vi "Instrument.Template.AppLauncher.vi"(8 "error in":errorcluster, 10 "Configuration Window? [T]":bool=TRUE, 11 "Debug Mode? [F]":bool) -> (0 "error out":errorcluster)   [LabVIEW 2019, in "Instrument.Template.lvclass"]
uses:
  Instrument.Template.lvclass
  <vilib>/JKI/JKI SMO/SMO/Typedefs/SMOState --Enum.ctl
  <userlib>/LevyLab/Levylab Instruments/SMOs/Instrument/Instrument.lvclass
  C:/Program Files (x86)/National Instruments/LabVIEW 2019/vi.lib/JKI/JKI SMO/SMO/SMO.lvclass
  <userlib>/LevyLab/Levylab Instruments/SMOs/Instrument UI/Instrument UI.lvclass
  C:/Program Files (x86)/National Instruments/LabVIEW 2019/vi.lib/JKI/JKI SMO/SMO.UI/SMO.UI.lvclass
  Program Files (x86)/National Instruments/LabVIEW 2019/templates/JKI/JKI SMO/Instrument Framework/Templates/Instrument UI.Template/Instrument UI.Template.lvclass
  C:/Program Files (x86)/National Instruments/LabVIEW 2019/user.lib/LevyLab/Levylab Instruments/SMOs/Instrument UI/Instrument UI.lvclass
  C:/Program Files (x86)/National Instruments/LabVIEW 2019/user.lib/LevyLab/Levylab Instruments/SMOs/Instrument/Instrument.lvclass
  <vilib>/JKI/JKI SMO/SMO/SMO.lvclass/SMO.ctl
  <vilib>/JKI/JKI SMO/SMO/Private/ReftoDVR--SMO.vi
  <vilib>/JKI/JKI SMO/SMO/SMO.lvclass
  <vilib>/JKI/JKI SMO/SMO.UI/SMO.UI.lvclass
panel:
  in  "Splash Status":string="Push Start to Start..." caption="String"
  in  "Start":bool=TRUE
  in  "Stop":bool=TRUE
  out "UI SMO State":T1=enum."Stopped"
  out "SMO State":T1
  # "Example Instrument SMO Test Launcher"
  # "For instructions on how to use the JKI State Machine Objects, examples and video tutorials, visit:\nhttp://jki.net/state-machine-objects/\n\nJKI State Machine Objects™\nhttp://jki.net/state-machine-objects/\nCopyright (C) 2005-2015, JKI <info@jki.net>\nALL RIGHTS RESERVED"
  # "Starting Example Instrument..."
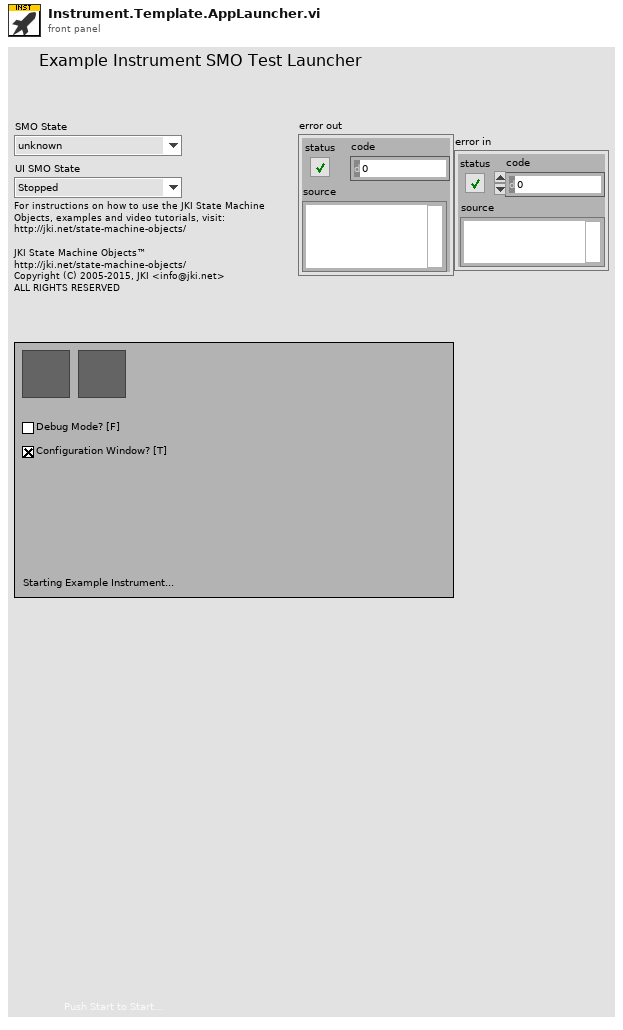
[diagram p1: front panel]
types:
  T1 = typedef "SMO.lvclass/SMOState --Enum.ctl" = enum16{"unknown", "Created", "Started", "Stopped"}
  T2 = enum32{"Invalid", "Standard", "Closed", "Hidden", "Minimized", "Maximized"}
  T3 = enum32{"invalid app kind", "Development System", "Run Time System", "Student Edition", "Embedded LabVIEW", "Evaluation", "Custom"}
  T4 = cluster{"Core":cluster{"Current VI Reference":refnum<vi>, "Close Panel on Exit?":bool}, "Instrument.lvclass":refnum<class "Instrument.lvclass">, "Instrument UI.lvclass":refnum<class "Instrument UI.lvclass">}
  T5 = cluster{"Current VI Reference":refnum<vi>, "Close Panel on Exit?":bool}
  T6 = typedef "SMO.lvclass/Public Events.ctl" = cluster{"Error":refnum<user-event>, "State":refnum<user-event>, "Reserve State":refnum<user-event>}
  T7 = cluster{"Event Registration Refnum":refnum<event-registration>, "Event Registration Refnum":refnum<event-registration>}
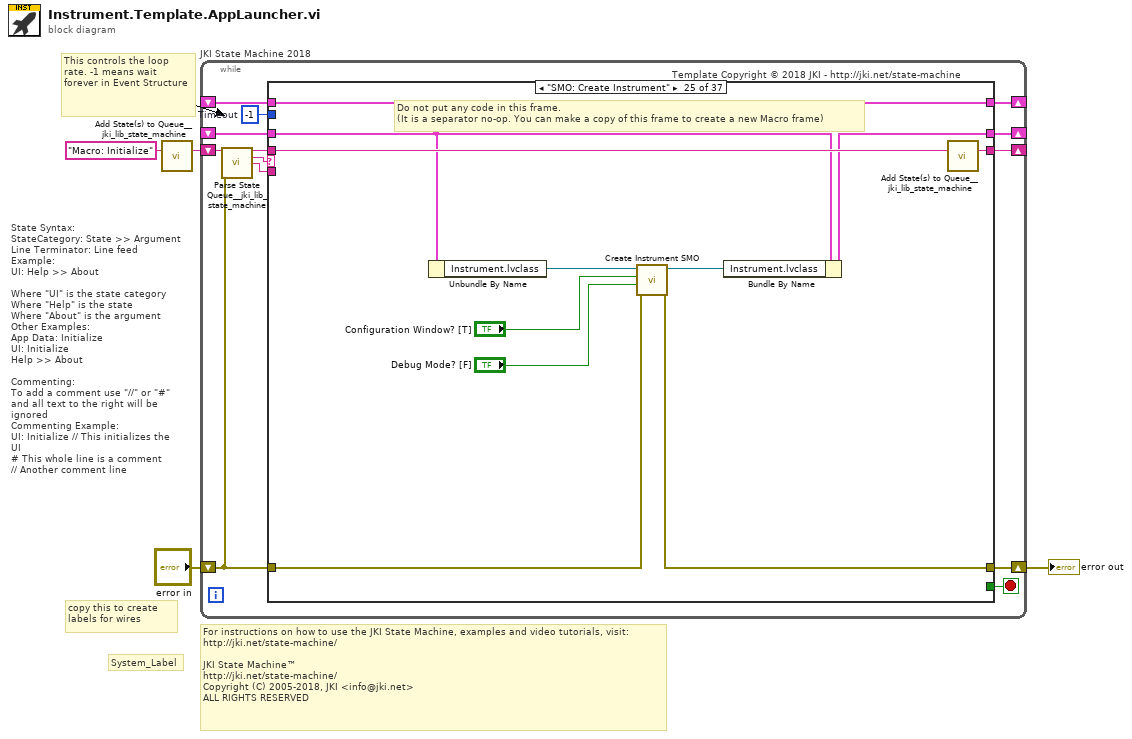
[diagram p0: block diagram]
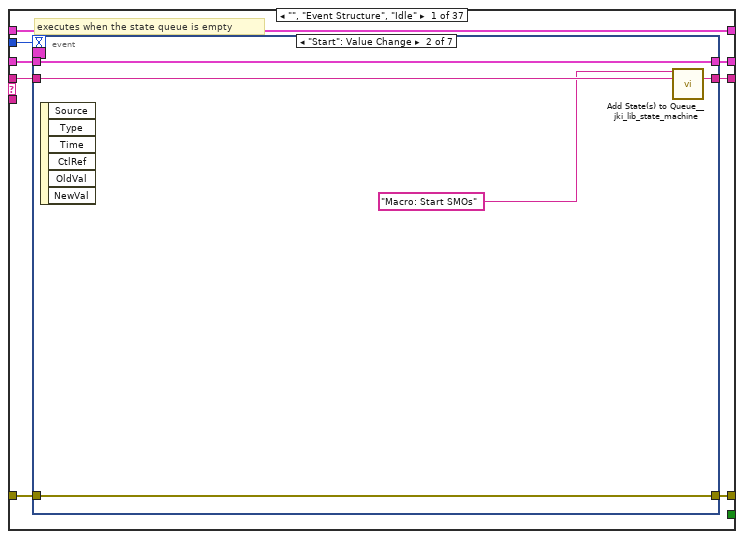
[diagram p2: hidden frame]
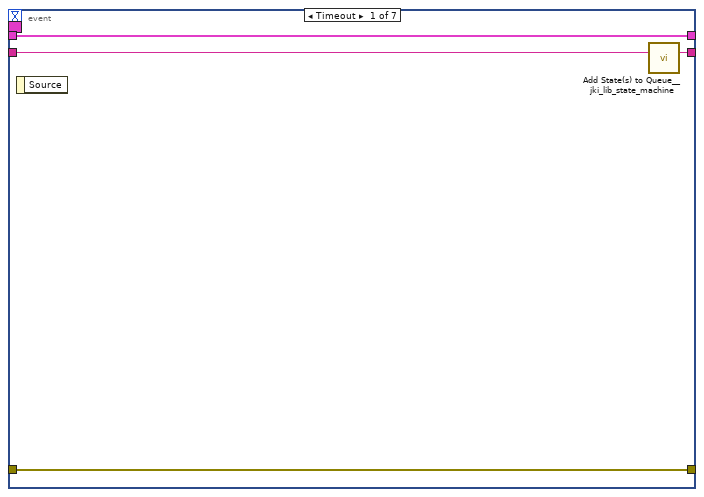
[diagram p3: hidden frame]
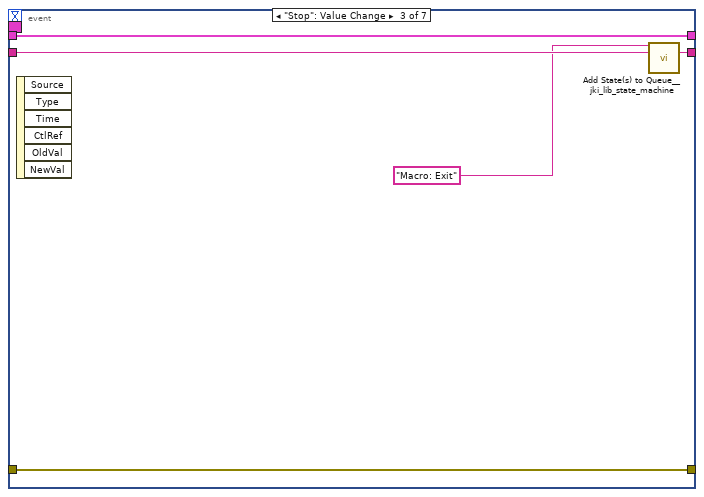
[diagram p4: hidden frame]
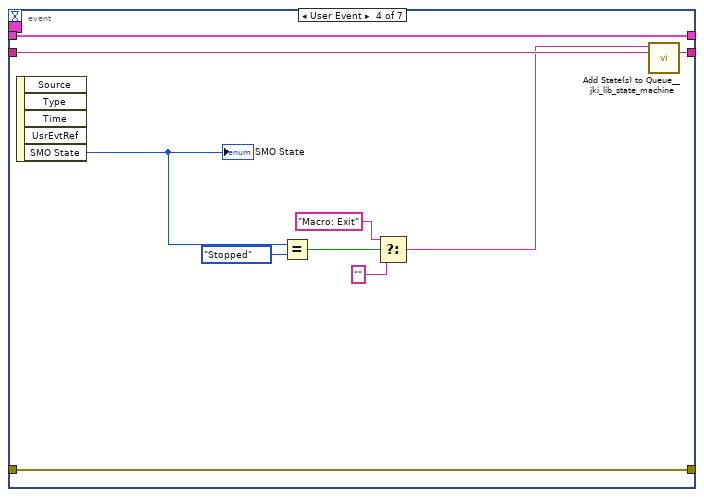
[diagram p5: hidden frame]
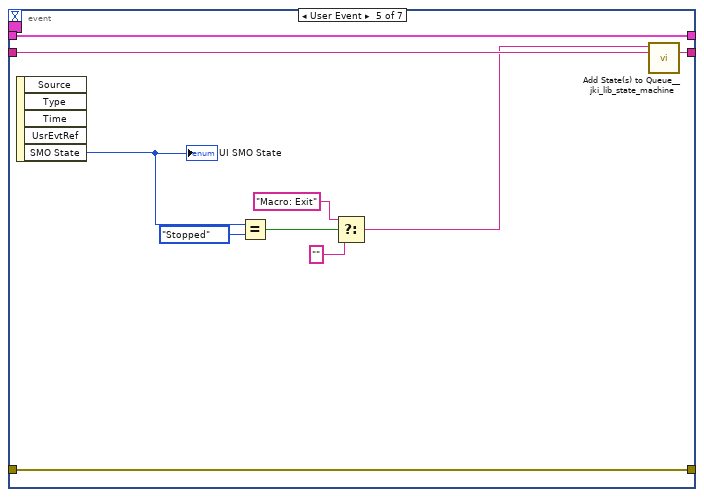
[diagram p6: hidden frame]
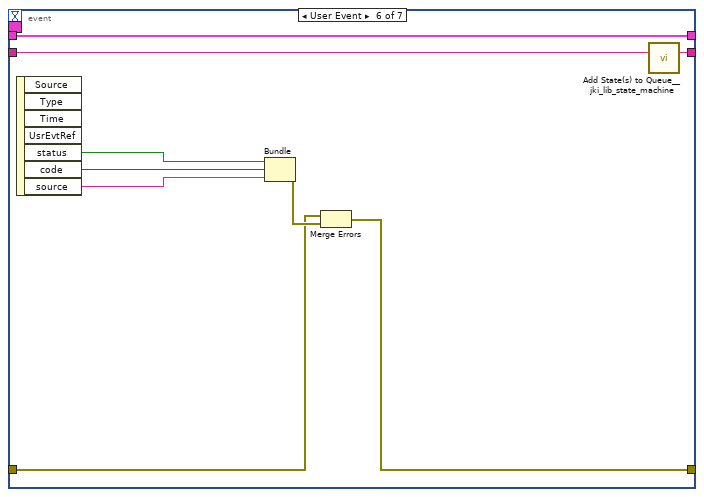
[diagram p7: hidden frame]
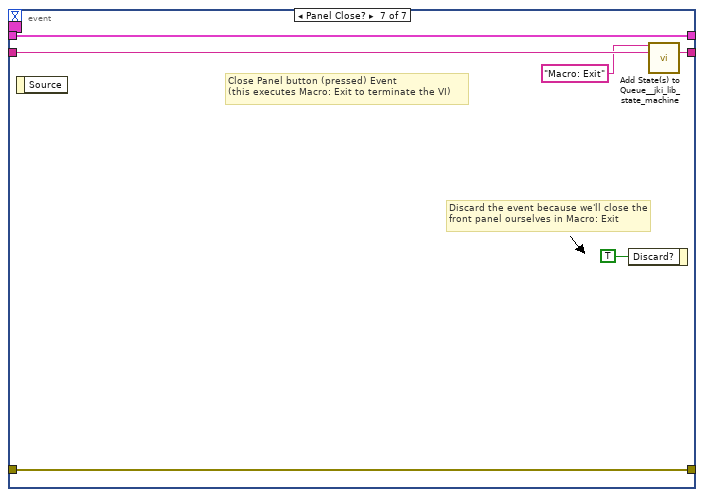
[diagram p8: hidden frame]
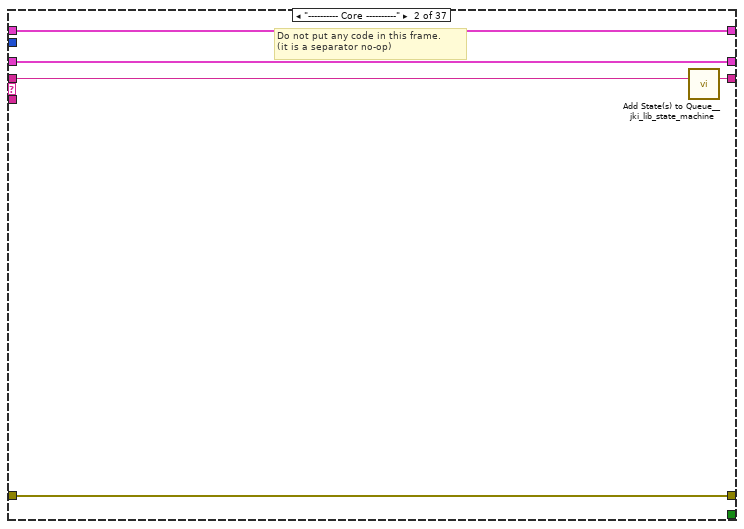
[diagram p9: hidden frame]
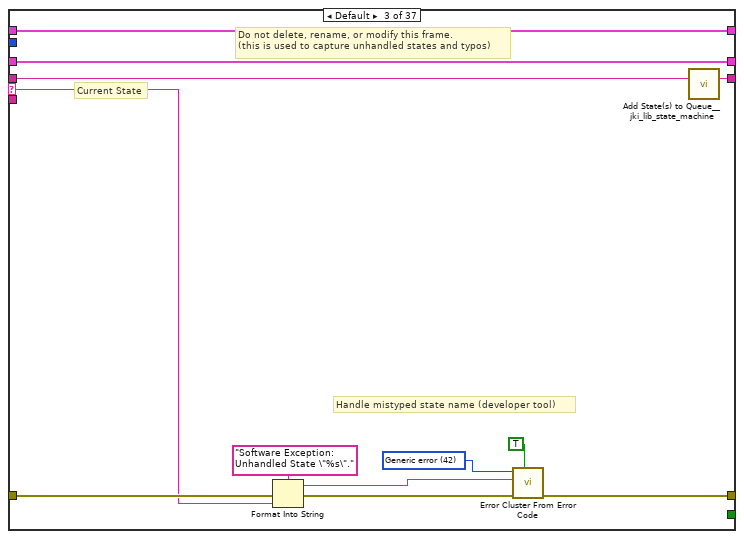
[diagram p10: hidden frame]
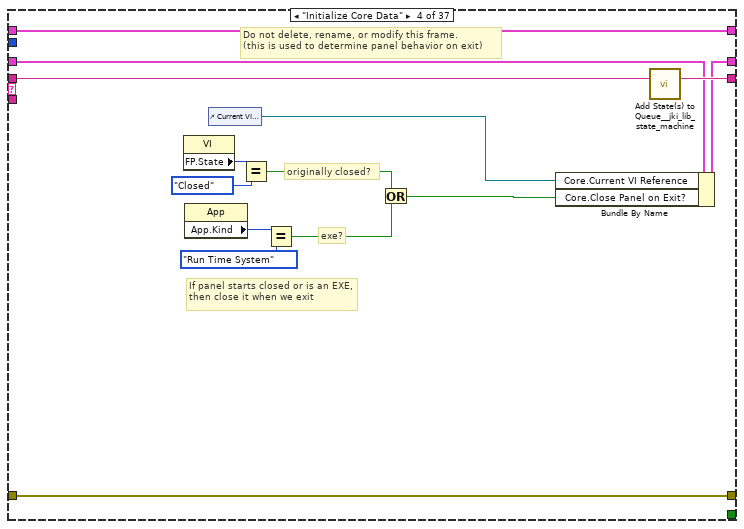
[diagram p11: hidden frame]
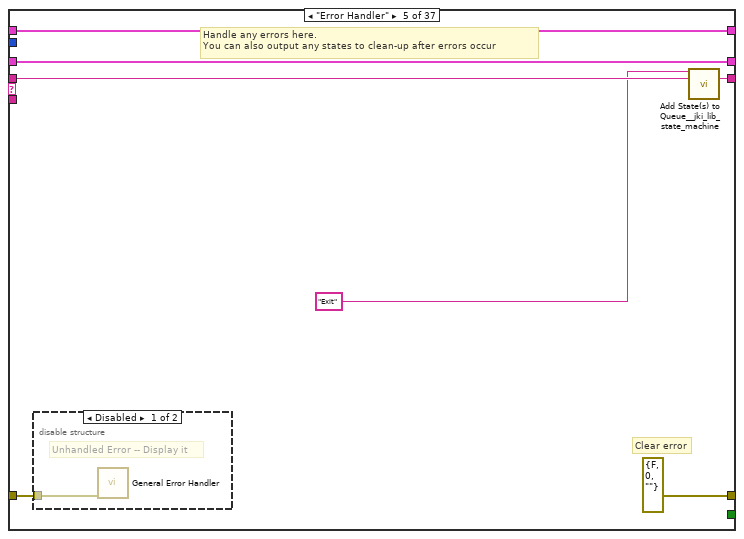
[diagram p12: hidden frame]
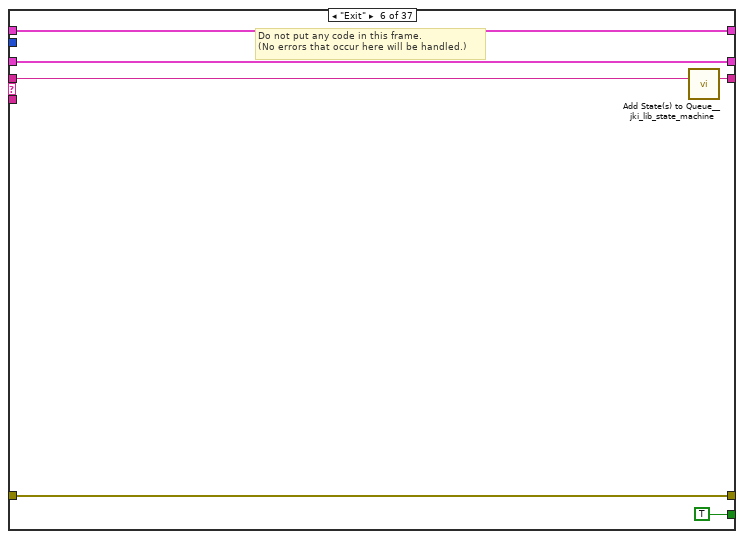
[diagram p14: hidden frame]
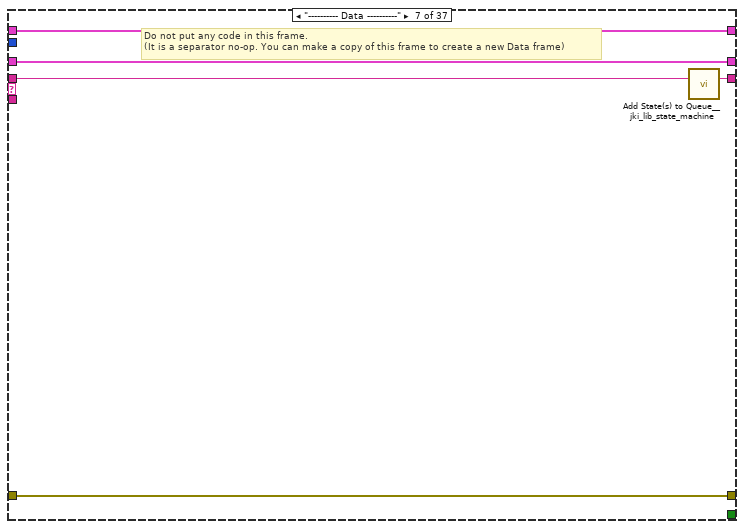
[diagram p15: hidden frame]
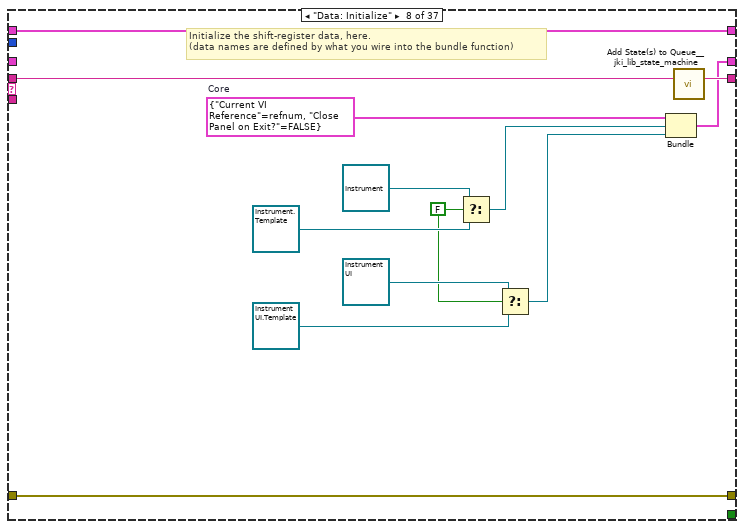
[diagram p16: hidden frame]
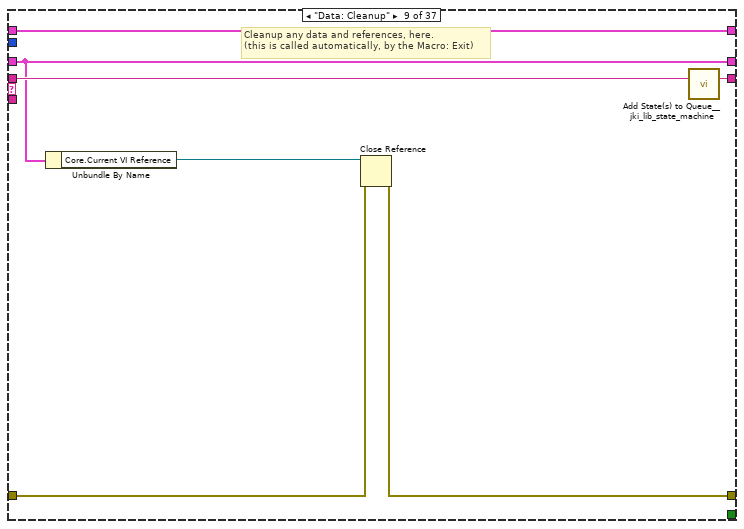
[diagram p17: hidden frame]
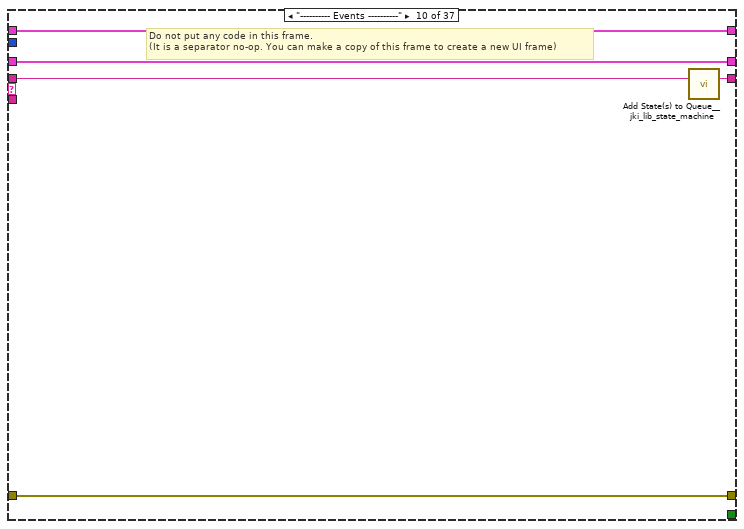
[diagram p18: hidden frame]
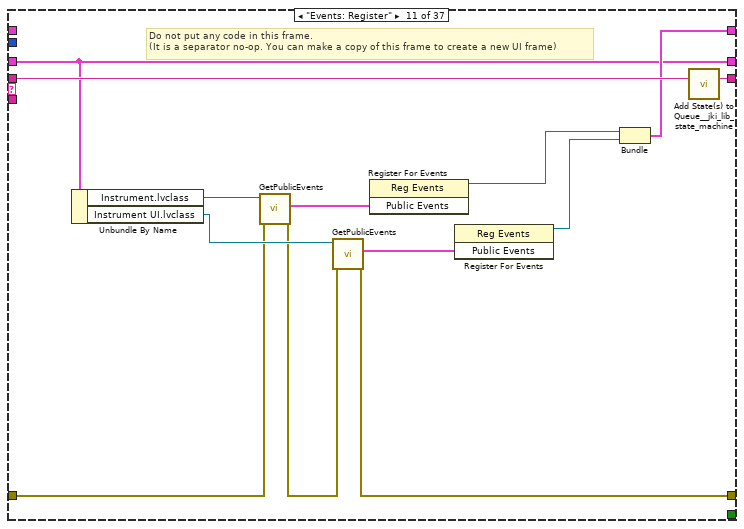
[diagram p19: hidden frame]
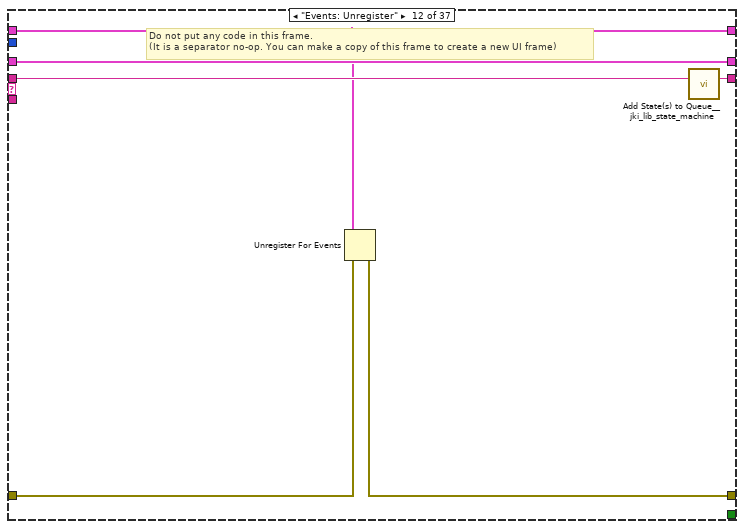
[diagram p20: hidden frame]
diagram:
  # "For instructions on how to use the JKI State Machine, examples and video tutorials, visit:\nhttp://jki.net/state-machine/\n\nJKI State Machine™\nhttp://jki.net/state-machine/\nCopyright (C) 2005-2018, JKI <info@jki.net>\nALL RIGHTS RESERVED"
  # "State Syntax:\nStateCategory: State >> Argument\nLine Terminator: Line feed\nExample:\nUI: Help >> About\n\nWhere \"UI\" is the state category\nWhere \"Help\" is the state\nWhere \"About\" is the argument\nOther Examples:\nApp Data: Initialize\nUI: Initialize\nHelp >> About\n\nCommenting:\nTo add a comment use \"//\" or \"#\" and all text to the right will be ignored\nCommenting Example:\nUI: Initialize // This initializes the UI\n# This whole line is a comment\n// Another comment line"
  # "copy this to create labels for wires"
  # "This controls the loop rate. -1 means wait forever in Event Structure"
  # "System_Label"
  n1 = call <vilib>:"Add State(s) to Queue__jki_lib_state_machine.vi"("State(s) in (\"\")"="Macro: Initialize") -> ("States Out"=w4:string)  [unwired: 14 in]
  n2 = while "JKI State Machine 2018" {
    shift-right: [w11] -> _
    shift-left: _ -> [w6]
    shift-right: [w14] -> w2
    shift-left: "error in" -> [w9]
    shift-right: [w13] -> _
    shift-left: w4 -> [w15]
    shift-right: [w8] -> _
    shift-left: _ -> [w7]
    stop <- w12 stop-if-true
    w10 = -1  # Timeout
    # "Template Copyright © 2018 JKI - http://jki.net/state-machine"
    n3 = call <vilib>:"Parse State Queue__jki_lib_state_machine.vi"("State Queue"=w15, "Error In (no error)"=w9) -> ("Remaining States"=w17:string, "Current State"=w5:string, "Arguments"=w16:string)  [unwired: 11 in]
    n4 = case shown="\"SMO: Create Instrument\"" w5 {
      selector: w5 -> [_ _ w81 _ _ _ _ _ _ _ _ _ _ _ _ _ _ _ _ _ _ _ _ _ _ _ _ _ _ _ _ _ _ _ _ _ _]
      tunnel: w17 -> [w25 w79 w85 w105 w112 w119 w124 w137 w144 w149 w162 w168 w173 w179 w186 w198 w276 w281 w286 w292 w298 w304 w316 w321 w332 w341 w351 w358 w369 w384 w399 w414 w429 w444 w453 w460 w465]
      tunnel: w16 -> [_ _ _ _ _ _ _ _ _ _ _ _ _ _ w181 w192 _ _ _ _ _ _ _ _ _ _ _ _ _ _ _ _ _ _ _ w457 _]
      tunnel: [w22 w77 w87 w102 errorcluster {"status"=FALSE, "code"=0, "source"=""} ("error out") w116 w122 w132 w140 w147 w151 w163 w171 w174 w182 w195 w266 w279 w284 w290 w296 w302 w314 w319 w328 w333 w342 w352 w365 w380 w395 w411 w426 w441 w451 w455 w463] -> w14
      tunnel: w9 -> [w21 w77 w86 w102 w108 w116 w122 w132 w141 w147 w153 w164 w171 w176 w183 w196 w267 w279 w284 w290 w296 w302 w314 w319 w329 w334 w343 w353 w362 w376 w392 w409 w424 w437 w451 w456 w463]
      tunnel: [w24 w78 w84 w104 w111 w118 w123 w136 w143 w148 w161 w167 w172 w178 w185 w197 w275 w280 w285 w291 w297 w303 w315 w320 w331 w340 w350 w357 w368 w383 w398 w413 w428 w443 w452 w459 w464] -> w13
      tunnel: [_ _ _ _ _ TRUE _ _ _ _ _ _ _ _ _ _ _ _ _ _ _ _ _ _ _ _ _ _ _ _ _ _ _ _ _ _ _] -> w12
      tunnel: [w20 w76 w83 w103 w109 w117 w121 w135 w139 w146 w156 w166 w170 w177 w184 w194 w264 w278 w283 w289 w295 w301 w313 w318 w327 w336 w347 w355 w366 w381 w396 w410 w425 w440 w450 w458 w462] -> w11
      tunnel: w10 -> [w19 _ _ _ _ _ _ _ _ _ _ _ _ _ _ _ _ _ _ _ _ _ _ _ _ _ _ _ _ _ _ _ _ _ _ _ _]
      tunnel: [w18 w75 w80 w92 w106 w114 w120 w133 w138 w145 w159 w165 w169 w175 w180 w191 w265 w277 w282 w287 w294 w300 w307 w317 w330 w339 w349 w356 w367 w382 w397 w412 w427 w442 w449 w454 w461] -> w8
      tunnel: w7 -> [w18 w75 w80 w92 w106 w114 w120 w133 w138 w145 _ w165 w169 w175 w180 w191 w265 w277 w282 w287 w294 w300 w307 w317 w330 w339 w349 w356 w367 w382 w397 w412 w427 w442 w449 w454 w461]
      tunnel: w6 -> [w23 w76 w83 w98 w109 w117 w121 _ w139 w146 w156 w166 w170 w177 w184 w194 w264 w278 w283 w289 w295 w301 w313 w318 w325 w337 w348 w355 w366 w381 w396 w410 w425 w440 w450 w458 w462]
      frame "", "Event Structure", "Idle" {
        # "executes when the state queue is empty"
        n5 = event shown="[1] \"Start\": Value Change" {
          selector: w18 -> [_ _ _ _ _ _ _]
          dyn-events: _ -> [_ _ _ _ _ _ _]
          timeout: w19 -> [_ _ _ _ _ _ _]
          tunnel: w25 -> [w29 w34 w39 w49 w59 w68 w74]
          tunnel: [w28 w33 w38 w48 w58 w67 w73] -> w24
          tunnel: w23 -> [w26 w31 w36 w46 w56 w66 w71]
          tunnel: [w27 w32 w37 w47 w57 w63 w72] -> w22
          tunnel: w21 -> [w27 w32 w37 w47 w57 w64 w72]
          tunnel: [w26 w31 w36 w46 w56 w66 w71] -> w20
          event Timeout {
            n6 = event-data() -> ()  [unwired: 1 in, 1 out]
            n7 = call <vilib>:"Add State(s) to Queue__jki_lib_state_machine.vi"("State(s) in (\"\")"=w29) -> ("States Out"=w28:string)  [unwired: 14 in]
          }
          event "Start": Value Change {
            n8 = event-data() -> ()  [unwired: 1 in, 6 out]
            n9 = call <vilib>:"Add State(s) to Queue__jki_lib_state_machine.vi"("State(s) in Front (\"\")"="Macro: Start SMOs" ("State(s) in Front (\"\")"), "State(s) in (\"\")"=w34) -> ("States Out"=w33:string)  [unwired: 13 in]
          }
          event "Stop": Value Change {
            n10 = event-data() -> ()  [unwired: 1 in, 6 out]
            n11 = call <vilib>:"Add State(s) to Queue__jki_lib_state_machine.vi"("State(s) in Front (\"\")"="Macro: Exit" ("State(s) in Front (\"\")"), "State(s) in (\"\")"=w39) -> ("States Out"=w38:string)  [unwired: 13 in]
          }
          event User Event {
            n12 = event-data() -> ("SMO State"=w41:T1)  [unwired: 1 in, 4 out]
            "SMO State" <- w41
            n13 = Equal?(x=w41, y=SMOState_--Enum."Stopped") -> (x = y?=w44:bool)
            n14 = Select(t="Macro: Exit", s=w44, f="" ("State(s) in Front (\"\")")) -> (s? t:f=w40:string)
            n15 = call <vilib>:"Add State(s) to Queue__jki_lib_state_machine.vi"("State(s) in Front (\"\")"=w40, "State(s) in (\"\")"=w49) -> ("States Out"=w48:string)  [unwired: 13 in]
          }
          event User Event {
            n16 = event-data() -> ("SMO State"=w50:T1)  [unwired: 1 in, 4 out]
            "UI SMO State" <- w50
            n17 = Equal?(x=w50, y=SMOState_--Enum."Stopped") -> (x = y?=w54:bool)
            n18 = Select(t="Macro: Exit", s=w54, f="" ("State(s) in Front (\"\")")) -> (s? t:f=w52:string)
            n19 = call <vilib>:"Add State(s) to Queue__jki_lib_state_machine.vi"("State(s) in Front (\"\")"=w52, "State(s) in (\"\")"=w59) -> ("States Out"=w58:string)  [unwired: 13 in]
          }
          event User Event {
            n20 = event-data() -> ("status"=w60:bool, "code"=w62:i32, "source"=w61:string)  [unwired: 1 in, 4 out]
            n21 = Bundle("status"=w60, "code"=w62, "source"=w61) -> (w65:errorcluster)  [unwired: 1 in]
            n22 = Merge Errors(w64, w65) -> (w63:errorcluster)
            n23 = call <vilib>:"Add State(s) to Queue__jki_lib_state_machine.vi"("State(s) in (\"\")"=w68) -> ("States Out"=w67:string)  [unwired: 14 in]
          }
          event Panel Close? {
            # "Discard the event because we'll close the front panel ourselves in Macro: Exit"
            # "Close Panel button (pressed) Event\n(this executes Macro: Exit to terminate the VI)"
            n24 = event-data() -> ()  [unwired: 1 in, 1 out]
            n25 = event-data("Discard?"=TRUE) -> ()  [unwired: 1 in, 1 out]
            n26 = call <vilib>:"Add State(s) to Queue__jki_lib_state_machine.vi"("State(s) in Front (\"\")"="Macro: Exit", "State(s) in (\"\")"=w74) -> ("States Out"=w73:string)  [unwired: 13 in]
          }
        }
      }
      frame "---------- Core ----------" {
        # "Do not put any code in this frame.\n(it is a separator no-op)"
        n27 = call <vilib>:"Add State(s) to Queue__jki_lib_state_machine.vi"("State(s) in (\"\")"=w79) -> ("States Out"=w78:string)  [unwired: 14 in]
      }
      frame Default {
        w90 = 42 items=["No error", "Argument error", "Memory is full", "Out of zone", "End of file", "File already open", "Generic file I/O error", "File not found", "File permission error", "Disk is full", "Duplicate path", "Too many files open", "System feature not enabled", "Resource file not found", "Cannot add resource", "Resource not found", "Image not found", "Image memory error", "Pen does not exist", "Config type invalid", "Config token not found", "Config parse error", "Config memory error", "Bad external code format", "Bad external code offset", "External code not present", "Null window", "Destroy window error", "Null menu", "Print aborted", "Bad print record", "Print driver error", "Windows error during printing", "Memory error during printing", "Print dialog error", "Generic print error", "Invalid device refnum", "Device not found", "Device parameter error", "Device unit error", "Cannot open device", "Device call aborted", "Generic error", "Cancelled by user", "Object ID too low", "Object ID too high", "Object not in heap", "Unknown heap", "Unknown object (invalid DefProc)", "Unknown object (DefProc not in table)", "Message out of range", "Invalid (null) method", "Unknown message", "Manager call not supported", "Bad address", "Network operation in progress", "Network operation timed out", "Connection is busy", "Network attribute not supported", "Network error", "Address in use", "System out of memory", "Connection aborted", "Connection refused", "Not connected", "Already connected", "Connection closed", "Initialization error (interapplication manager)", "Bad occurrence", "Wait on unbound occurrence handler", "Occurrence queue overflow", "Datalog type conflict", "Unused", "Unrecognized type (interapplication manager)", "Memory corrupt", "Failed to make temporary DLL", "Old CIN version", "Drag socket not found", "Failed to load drop-object", "Failed to register OLE object", "Failed to release OLE object", "Format specifier type mismatch", "Unknown format specifier", "Too few format specifiers", "Too many format specifiers", "Scan failed", "Newer CIN version", "Error converting to variant", "Runtime menu error", "Password tampered", "Variant attribute not found", "Incompatible variant data type", "Event data is not available", "Event Store is not present", "Occurrence is not found", "Event Queue is not created", "Event info is not available", "Refnum passed is NULL", "Error retrieving Class GUID", "Error retrieving CoClass GUID", "Error retrieving TypeLib GUID.", "Bad built application magic bytes.", "Specific driver is different from the specific driver associated with the Logical Name.", "There is no session opened to the class driver.", "Max Error", "MAX - Error with config objects", "MAX - Error loading configuration", "MAX - Group not supported"]
        # "Current State"
        # "Do not delete, rename, or modify this frame.\n(this is used to capture unhandled states and typos)"
        # "Handle mistyped state name (developer tool)"
        n28 = Format Into String(format string="Software Exception: Unhandled State \"%s\"." ("message"), error in=w86, w81) -> (resulting string=w89:string, error out=w88:errorcluster)  [unwired: 1 in]
        n29 = call <vilib>:"Error Cluster From Error Code.vi"("show call chain? (False)"=TRUE, "error in (no error)"=w88, "error message (\"\")"=w89, "error code (0)"=w90) -> ("error out"=w87:errorcluster)  [unwired: 5 in]
        n30 = call <vilib>:"Add State(s) to Queue__jki_lib_state_machine.vi"("State(s) in (\"\")"=w85) -> ("States Out"=w84:string)  [unwired: 14 in]
      }
      frame "Initialize Core Data" {
        # "Do not delete, rename, or modify this frame.\n(this is used to determine panel behavior on exit)"
        # "originally closed?"
        # "exe?"
        # "If panel starts closed or is an EXE, then close it when we exit"
        n31 = property class="VI"() -> ("FP.State"=w95:T2)  [unwired: 2 in, 2 out]
        n32 = property class="App"() -> ("App.Kind"=w101:T3)  [unwired: 2 in, 2 out]
        n33 = control-ref of="Current VI Reference"() -> (w96:refnum<vi>)
        n34 = Equal?(x=w95, y=T2."Closed" ("Front Panel Window:State")) -> (x = y?=w93:bool)
        n35 = Equal?(x=w101, y=T3."Run Time System" ("Application:Kind")) -> (x = y?=w99:bool)
        n36 = Or(x=w93, y=w99) -> (x .or. y?=w97:bool)
        n37 = Bundle By Name(cluster=w98, "Core.Current VI Reference"=w96, "Core.Close Panel on Exit?"=w97) -> (w103:T4)
        n38 = call <vilib>:"Add State(s) to Queue__jki_lib_state_machine.vi"("State(s) in (\"\")"=w105) -> ("States Out"=w104:string)  [unwired: 14 in]
      }
      frame "Error Handler" {
        # "Handle any errors here.\nYou can also output any states to clean-up after errors occur"
        # "Clear error"
        n39 = disable-structure shown="Disabled" {
          disable-tunnel: w108 -> [w113 _]
          frame Disabled {
            # "Unhandled Error -- Display it"
            n40 = call <vilib>:"General Error Handler.vi"("error in (no error)"=w113) -> ()  [unwired: 10 in, 5 out]
          }
          frame Enabled {
          }
        }
        n41 = call <vilib>:"Add State(s) to Queue__jki_lib_state_machine.vi"("State(s) in Front (\"\")"="Exit", "State(s) in (\"\")"=w112) -> ("States Out"=w111:string)  [unwired: 13 in]
      }
      frame "Exit" {
        # "Do not put any code in this frame.\n(No errors that occur here will be handled.)"
        n42 = call <vilib>:"Add State(s) to Queue__jki_lib_state_machine.vi"("State(s) in (\"\")"=w119) -> ("States Out"=w118:string)  [unwired: 14 in]
      }
      frame "---------- Data ----------" {
        # "Do not put any code in this frame.\n(It is a separator no-op. You can make a copy of this frame to create a new Data frame)"
        n43 = call <vilib>:"Add State(s) to Queue__jki_lib_state_machine.vi"("State(s) in (\"\")"=w124) -> ("States Out"=w123:string)  [unwired: 14 in]
      }
      frame "Data: Initialize" {
        w125 = FALSE ("s")
        w134 = T5 {"Current VI Reference"=refnum, "Close Panel on Exit?"=FALSE}  # Core
        # "Initialize the shift-register data, here.\n(data names are defined by what you wire into the bundle function)"
        n44 = Select(t=refnum<class "Instrument.lvclass"> refnum ("Instrument.lvclass"), s=w125, f=refnum<class "Instrument.Template.lvclass"> refnum ("Example.lvclass")) -> (s? t:f=w127:refnum<class "Instrument.lvclass">)
        n45 = Select(t=refnum<class "Instrument UI.lvclass"> refnum ("Instrument UI.lvclass"), s=w125, f=refnum<class "Instrument UI.Template.lvclass"> refnum ("Example UI.lvclass")) -> (s? t:f=w126:refnum<class "Instrument UI.lvclass">)
        n46 = Bundle("Core"=w134, "Instrument.lvclass"=w127, "Instrument UI.lvclass"=w126) -> (w135:T4)  [unwired: 1 in]
        n47 = call <vilib>:"Add State(s) to Queue__jki_lib_state_machine.vi"("State(s) in (\"\")"=w137) -> ("States Out"=w136:string)  [unwired: 14 in]
      }
      frame "Data: Cleanup" {
        # "Cleanup any data and references, here.\n(this is called automatically, by the Macro: Exit)"
        n48 = Unbundle By Name(w139) -> ("Core.Current VI Reference"=w142:refnum<vi>)
        n49 = Close Reference(reference=w142, error in (no error)=w141) -> (error out=w140:errorcluster)
        n50 = call <vilib>:"Add State(s) to Queue__jki_lib_state_machine.vi"("State(s) in (\"\")"=w144) -> ("States Out"=w143:string)  [unwired: 14 in]
      }
      frame "---------- Events ----------" {
        # "Do not put any code in this frame.\n(It is a separator no-op. You can make a copy of this frame to create a new UI frame)"
        n51 = call <vilib>:"Add State(s) to Queue__jki_lib_state_machine.vi"("State(s) in (\"\")"=w149) -> ("States Out"=w148:string)  [unwired: 14 in]
      }
      frame "Events: Register" {
        # "Do not put any code in this frame.\n(It is a separator no-op. You can make a copy of this frame to create a new UI frame)"
        n52 = Unbundle By Name(w156) -> ("Instrument.lvclass"=w155:refnum<class "Instrument.lvclass">, "Instrument UI.lvclass"=w154:refnum<class "Instrument UI.lvclass">)
        n53 = call <vilib>:"GetPublicEvents.vi"("error in (no error)"=w153, "SMO"=w155) -> ("error out"=w152:errorcluster, "Public Events"=w157:T6)  [unwired: 7 in, 1 out]
        n54 = call <vilib>:"GetPublicEvents.vi"("error in (no error)"=w152, "SMO"=w154) -> ("error out"=w151:errorcluster, "Public Events"=w158:T6)  [unwired: 7 in, 1 out]
        n55 = register-events(w157) -> (reference out=w160:refnum<event-registration>)  [unwired: 2 in, 1 out]
        n56 = register-events(w158) -> (reference out=w150:refnum<event-registration>)  [unwired: 2 in, 1 out]
        n57 = Bundle("Event Registration Refnum"=w160, "Event Registration Refnum"=w150) -> (w159:T7)  [unwired: 1 in]
        n58 = call <vilib>:"Add State(s) to Queue__jki_lib_state_machine.vi"("State(s) in (\"\")"=w162) -> ("States Out"=w161:string)  [unwired: 14 in]
      }
      frame "Events: Unregister" {
        # "Do not put any code in this frame.\n(It is a separator no-op. You can make a copy of this frame to create a new UI frame)"
        n59 = Unregister For Events(event registration refnum=w165, error in=w164) -> (error out=w163:errorcluster)
        n60 = call <vilib>:"Add State(s) to Queue__jki_lib_state_machine.vi"("State(s) in (\"\")"=w168) -> ("States Out"=w167:string)  [unwired: 14 in]
      }
      frame "---------- UI ----------" {
        # "Do not put any code in this frame.\n(It is a separator no-op. You can make a copy of this frame to create a new UI frame)"
        n61 = call <vilib>:"Add State(s) to Queue__jki_lib_state_machine.vi"("State(s) in (\"\")"=w173) -> ("States Out"=w172:string)  [unwired: 14 in]
      }
      frame "UI: Initialize" {
        # "Initialize the User Interface, here.\n(this is called automatically, by the Macro: Init)"
        n62 = invoke on="Stop" class="Bool (strict)" method="Reinit To Default"() -> ()  [unwired: 3 in, 3 out]
        n63 = invoke on="error out" class="Clust (strict)" method="Reinit To Default"() -> ()  [unwired: 3 in, 3 out]
        n64 = invoke on="SMO State 2" class="Enum (strict)" method="Reinit To Default"() -> ()  [unwired: 3 in, 3 out]
        n65 = invoke on="Start" class="Bool (strict)" method="Reinit To Default"() -> ()  [unwired: 3 in, 3 out]
        n66 = call <userlib>:"Fit VI window to Largest Dec__ogtk.vi"("error in (no error)"=w176) -> ("error out"=w174:errorcluster)  [unwired: 5 in, 1 out]
        n67 = call <vilib>:"Add State(s) to Queue__jki_lib_state_machine.vi"("State(s) in (\"\")"=w179) -> ("States Out"=w178:string)  [unwired: 14 in]
      }
      frame "UI: Cursor Set" {
        # "Argument"
        # "Set and Unset Cursor Busy.\n(Usage: \"UI: Cursor Set >> Busy|Idle\")"
        n68 = case shown="\"Busy\"" w181 {
          tunnel: w183 -> [w188 w190]
          tunnel: [w187 w189] -> w182
          frame "Idle", Default {
            n69 = call <vilib>:"Unset Busy.vi"("error in (no error)"=w188) -> ("error out"=w187:errorcluster)  [unwired: 10 in]
          }
          frame "Busy" {
            n70 = call <vilib>:"Set Busy.vi"("error in (no error)"=w190) -> ("error out"=w189:errorcluster)  [unwired: 9 in, 1 out]
          }
        }
        n71 = call <vilib>:"Add State(s) to Queue__jki_lib_state_machine.vi"("State(s) in (\"\")"=w186) -> ("States Out"=w185:string)  [unwired: 14 in]
      }
      frame "UI: Front Panel State" {
        # "Argument"
        # "Set Front Panel Open or Closed\n(Usage: \"UI: Front Panel State >> Open|Close\")"
        n72 = Unbundle By Name(w194) -> ("Core.Current VI Reference"=w193:refnum<vi>)
        n73 = case shown="\"Open\", \"Standard\", Default" w192 {
          tunnel: w196 -> [w204 w219 w230 w243 w256]
          tunnel: [w206 w220 w232 w245 w258] -> w195
          tunnel: w193 -> [w205 w217 w231 w244 w257]
          frame "Open", "Standard", Default {
            w199 = T2."Standard" ("State")
            n74 = property class="VI"(reference=w205, error in=w204) -> (reference out=w202:refnum<vi>, error out=w203:errorcluster, "FP.State"=w201:T2)
            n75 = Not Equal?(x=w201, y=w199) -> (x != y?=w200:bool)
            n76 = case shown="False" w200 {
              tunnel: [w210 w212] -> w206
              tunnel: w203 -> [w209 w212]
              tunnel: w202 -> [w208 _]
              tunnel: w199 -> [w207 _]
              frame True {
                n77 = invoke class="VI" method="FP.Open"(reference=w208, error in=w209, "Activate"=TRUE, "State"=w207) -> (error out=w210:errorcluster)  [unwired: 1 in, 4 out]
              }
              frame False {
              }
            }
          }
          frame "Close", "Closed" {
            n78 = property class="VI"(reference=w217, error in=w219) -> (reference out=w216:refnum<vi>, error out=w218:errorcluster, "FP.State"=w214:T2)
            n79 = Not Equal?(x=w214, y=T2."Closed" ("Front Panel Window:State")) -> (x != y?=w213:bool)
            n80 = case shown="True" w213 {
              tunnel: [w221 w224] -> w220
              tunnel: w218 -> [w221 w223]
              tunnel: w216 -> [_ w222]
              frame False {
              }
              frame True {
                n81 = invoke class="VI" method="FP.Close"(reference=w222, error in=w223) -> (error out=w224:errorcluster)  [unwired: 1 in, 2 out]
              }
            }
          }
          frame "Hidden", "Hide" {
            w225 = T2."Hidden" ("State")
            n82 = property class="VI"(reference=w231, error in=w230) -> (reference out=w228:refnum<vi>, error out=w229:errorcluster, "FP.State"=w227:T2)
            n83 = Not Equal?(x=w227, y=w225) -> (x != y?=w226:bool)
            n84 = case shown="True" w226 {
              tunnel: [w236 w237] -> w232
              tunnel: w229 -> [w235 w237]
              tunnel: w228 -> [w234 _]
              tunnel: w225 -> [w233 _]
              frame True {
                n85 = invoke class="VI" method="FP.Open"(reference=w234, error in=w235, "State"=w233) -> (error out=w236:errorcluster)  [unwired: 2 in, 4 out]
              }
              frame False {
              }
            }
          }
          frame "Minimize", "Minimized" {
            w238 = T2."Minimized" ("State")
            n86 = property class="VI"(reference=w244, error in=w243) -> (reference out=w241:refnum<vi>, error out=w242:errorcluster, "FP.State"=w240:T2)
            n87 = Not Equal?(x=w240, y=w238) -> (x != y?=w239:bool)
            n88 = case shown="True" w239 {
              tunnel: [w249 w250] -> w245
              tunnel: w242 -> [w248 w250]
              tunnel: w241 -> [w247 _]
              tunnel: w238 -> [w246 _]
              frame True {
                n89 = invoke class="VI" method="FP.Open"(reference=w247, error in=w248, "State"=w246) -> (error out=w249:errorcluster)  [unwired: 2 in, 4 out]
              }
              frame False {
              }
            }
          }
          frame "Maximize", "Maximized" {
            w251 = T2."Maximized" ("State")
            n90 = property class="VI"(reference=w257, error in=w256) -> (reference out=w254:refnum<vi>, error out=w255:errorcluster, "FP.State"=w253:T2)
            n91 = Not Equal?(x=w253, y=w251) -> (x != y?=w252:bool)
            n92 = case shown="True" w252 {
              tunnel: [w262 w263] -> w258
              tunnel: w255 -> [w261 w263]
              tunnel: w254 -> [w260 _]
              tunnel: w251 -> [w259 _]
              frame True {
                n93 = invoke class="VI" method="FP.Open"(reference=w260, error in=w261, "State"=w259) -> (error out=w262:errorcluster)  [unwired: 2 in, 4 out]
              }
              frame False {
              }
            }
          }
        }
        n94 = call <vilib>:"Add State(s) to Queue__jki_lib_state_machine.vi"("State(s) in (\"\")"=w198) -> ("States Out"=w197:string)  [unwired: 14 in]
      }
      frame "UI: Set Background Color" {
        # "Do not put any code in this frame.\n(It is a separator no-op. You can make a copy of this frame to create a new UI frame)"
        n95 = property class="VI"(error in=w267) -> (error out=w269:errorcluster, "Panel"=w270:refnum<vi>)  [unwired: 1 in, 1 out]
        n96 = property class="Pnl"(reference=w270, error in=w269) -> (error out=w268:errorcluster, "Panes[]"=w271:refnum<vi>[])  [unwired: 1 out]
        n97 = Index Array(array=w271, index=0) -> (element=w273:refnum<vi>)
        n98 = property class="Pane"(reference=w273, error in=w268, "PaneColor"=u32 16777238 ("Color Box")) -> (error out=w266:errorcluster)  [unwired: 1 out]
        n99 = call <vilib>:"Add State(s) to Queue__jki_lib_state_machine.vi"("State(s) in (\"\")"=w276) -> ("States Out"=w275:string)  [unwired: 14 in]
      }
      frame "UI: Exit" {
        # "Do not put any code in this frame.\n(It is a separator no-op. You can make a copy of this frame to create a new UI frame)"
        n100 = invoke on="Start" class="Bool (strict)" method="Reinit To Default"() -> ()  [unwired: 3 in, 3 out]
        n101 = invoke on="Stop" class="Bool (strict)" method="Reinit To Default"() -> ()  [unwired: 3 in, 3 out]
        n102 = call <vilib>:"Add State(s) to Queue__jki_lib_state_machine.vi"("State(s) in (\"\")"=w281) -> ("States Out"=w280:string)  [unwired: 14 in]
      }
      frame "---------- Macro ----------" {
        # "Do not put any code in this frame.\n(It is a separator no-op. You can make a copy of this frame to create a new Macro frame)"
        n103 = call <vilib>:"Add State(s) to Queue__jki_lib_state_machine.vi"("State(s) in (\"\")"=w286) -> ("States Out"=w285:string)  [unwired: 14 in]
      }
      frame "Macro: Initialize" {
        # "Initialization Macro\n(This is called once, when the VI starts)"
        n104 = call <vilib>:"Add State(s) to Queue__jki_lib_state_machine.vi"("State(s) in Front (\"\")"="Data: Initialize\nInitialize Core Data\n//Events: Register\nUI: Initialize\nUI: Front Panel State >> Open\nUI: Set Background Color\nSplash: Set Status >> Push Start to Start...", "State(s) in (\"\")"=w292) -> ("States Out"=w291:string)  [unwired: 13 in]
      }
      frame "Macro: Start SMOs" {
        # "Do not put any code in this frame.\n(It is a separator no-op. You can make a copy of this frame to create a new Macro frame)"
        n105 = call <vilib>:"Add State(s) to Queue__jki_lib_state_machine.vi"("State(s) in Front (\"\")"="Splash: Set Status >> Starting Instrument...\nSMO: Create Instrument\nSMO: Create Instrument UI\nEvents: Register\nSMO: Start Instrument\nSplash: Set Status >> Instrument Process Started...\nSplash: Set Status >> Starting User Interface...\nSMO: Start Instrument UI\nUI: Front Panel State >> Hide\nSMO: Show Instrument UI" ("State(s) in Front (\"\")"), "State(s) in (\"\")"=w298) -> ("States Out"=w297:string)  [unwired: 13 in]
      }
      frame "Macro: Stop SMOs" {
        # "Do not put any code in this frame.\n(It is a separator no-op. You can make a copy of this frame to create a new Macro frame)"
        n106 = call <vilib>:"Add State(s) to Queue__jki_lib_state_machine.vi"("State(s) in Front (\"\")"="SMO: Stop Instrument\nSMO: Destroy Instrument\nSMO: Hide Instrument UI\nSMO: Stop Instrument UI\nSMO: Destroy Instrument UI" ("State(s) in Front (\"\")"), "State(s) in (\"\")"=w304) -> ("States Out"=w303:string)  [unwired: 13 in]
      }
      frame "Macro: Exit" {
        # "Exit Macro\n(This is called once, when the VI exits)"
        n107 = Unbundle By Name(w313) -> ("Core.Close Panel on Exit?"=w312:bool)
        n108 = Select(t="UI: Front Panel State >> Open", s=w312, f="") -> (s? t:f=w309:string)
        n109 = call <vilib>:"Add State(s) to Queue__jki_lib_state_machine.vi"("State(s) in Front (\"\")"="UI: Front Panel State >> Open\nUI: Exit", "State(s) in (\"\")"=w309, "State(s) at Back (\"\")"="Macro: Stop SMOs\nData: Cleanup\nEvents: Unregister\nExit") -> ("States Out"=w308:string)  [unwired: 12 in]
        n110 = call <vilib>:"Add State(s) to Queue__jki_lib_state_machine.vi"("State(s) in Front (\"\")"=w308, "State(s) in (\"\")"=w316) -> ("States Out"=w315:string)  [unwired: 13 in]
      }
      frame "---------- SMO ----------" {
        # "Do not put any code in this frame.\n(It is a separator no-op. You can make a copy of this frame to create a new Macro frame)"
        n111 = call <vilib>:"Add State(s) to Queue__jki_lib_state_machine.vi"("State(s) in (\"\")"=w321) -> ("States Out"=w320:string)  [unwired: 14 in]
      }
      frame "SMO: Create Instrument" {
        # "Do not put any code in this frame.\n(It is a separator no-op. You can make a copy of this frame to create a new Macro frame)"
        n112 = Unbundle By Name(w325) -> ("Instrument.lvclass"=w324:refnum<class "Instrument.lvclass">)
        n113 = call-dynamic "Create Instrument SMO.vi"("error in (no error)"=w329, "Debug Mode? [F]"="Debug Mode? [F]", "Configuration Window? [T]"="Configuration Window? [T]", "Instrument in"=w324) -> ("error out"=w328:errorcluster, "Instrument out"=w326:refnum<class "Instrument.lvclass">)  [unwired: 6 in]
        n114 = Bundle By Name(cluster=w325, "Instrument.lvclass"=w326) -> (w327:T4)
        n115 = call <vilib>:"Add State(s) to Queue__jki_lib_state_machine.vi"("State(s) in (\"\")"=w332) -> ("States Out"=w331:string)  [unwired: 14 in]
      }
      frame "SMO: Start Instrument" {
        # "Do not put any code in this frame.\n(It is a separator no-op. You can make a copy of this frame to create a new Macro frame)"
        n116 = Unbundle By Name(w337) -> ("Instrument.lvclass"=w338:refnum<class "Instrument.lvclass">)
        n117 = call <vilib>:"Start.vi"("error in (no error)"=w334, "SMO"=w338) -> ("error out"=w333:errorcluster, "SMO out"=w335:refnum<class "Instrument.lvclass">)  [unwired: 8 in]
        n118 = Bundle By Name(cluster=w337, "Instrument.lvclass"=w335) -> (w336:T4)
        n119 = call <vilib>:"Add State(s) to Queue__jki_lib_state_machine.vi"("State(s) in (\"\")"=w341) -> ("States Out"=w340:string)  [unwired: 14 in]
      }
      frame "SMO: Create Instrument UI" {
        # "Do not put any code in this frame.\n(It is a separator no-op. You can make a copy of this frame to create a new Macro frame)"
        n120 = Unbundle By Name(w348) -> ("Instrument UI.lvclass"=w346:refnum<class "Instrument UI.lvclass">, "Instrument.lvclass"=w345:refnum<class "Instrument.lvclass">)
        n121 = call <userlib>:"Create UI.vi"("error in (no error)"=w343, "Instrument in"=w345, "Instrument UI"=w346) -> ("error out"=w342:errorcluster, "Instrument UI out"=w344:refnum<class "Instrument UI.lvclass">)  [unwired: 7 in]
        n122 = Bundle By Name(cluster=w348, "Instrument UI.lvclass"=w344) -> (w347:T4)
        n123 = call <vilib>:"Add State(s) to Queue__jki_lib_state_machine.vi"("State(s) in (\"\")"=w351) -> ("States Out"=w350:string)  [unwired: 14 in]
      }
      frame "SMO: Start Instrument UI" {
        # "Do not put any code in this frame.\n(It is a separator no-op. You can make a copy of this frame to create a new Macro frame)"
        n124 = Unbundle By Name(w355) -> ("Instrument UI.lvclass"=w354:refnum<class "Instrument UI.lvclass">)
        n125 = call <vilib>:"Start.vi"("error in (no error)"=w353, "SMO"=w354) -> ("error out"=w352:errorcluster)  [unwired: 8 in, 1 out]
        n126 = call <vilib>:"Add State(s) to Queue__jki_lib_state_machine.vi"("State(s) in (\"\")"=w358) -> ("States Out"=w357:string)  [unwired: 14 in]
      }
      frame "SMO: Show Instrument UI" {
        # "Do not put any code in this frame.\n(It is a separator no-op. You can make a copy of this frame to create a new Macro frame)"
        n127 = Unbundle By Name(w366) -> ("Instrument UI.lvclass"=w364:refnum<class "Instrument UI.lvclass">)
        n128 = call <vilib>:"GetState.vi"("error in (no error)"=w362, "SMO"=w364) -> ("error out"=w360:errorcluster, "SMO State"=w359:T1, "SMO out"=w363:refnum<class "Instrument UI.lvclass">)  [unwired: 7 in]
        n129 = call <vilib>:"Clear Errors.vi"("error in (no error)"=w360) -> ("error out"=w361:errorcluster)  [unwired: 5 in, 1 out]
        n130 = case shown="\"Started\"" w359 {
          tunnel: [w370 w373] -> w365
          tunnel: w363 -> [_ w372]
          tunnel: w361 -> [w370 w371]
          frame Default {
          }
          frame "Started" {
            n131 = call <vilib>:"Show.vi"("error in (no error)"=w371, "SMO.UI"=w372) -> ("error out"=w373:errorcluster)  [unwired: 8 in, 1 out]
          }
        }
        n132 = call <vilib>:"Add State(s) to Queue__jki_lib_state_machine.vi"("State(s) in (\"\")"=w369) -> ("States Out"=w368:string)  [unwired: 14 in]
      }
      frame "SMO: Destroy Instrument" {
        # "Do not put any code in this frame.\n(It is a separator no-op. You can make a copy of this frame to create a new Macro frame)"
        n133 = Unbundle By Name(w381) -> ("Instrument.lvclass"=w379:refnum<class "Instrument.lvclass">)
        n134 = call <vilib>:"GetState.vi"("error in (no error)"=w376, "SMO"=w379) -> ("error out"=w375:errorcluster, "SMO State"=w378:T1, "SMO out"=w374:refnum<class "Instrument.lvclass">)  [unwired: 7 in]
        n135 = call <vilib>:"Clear Errors.vi"("error in (no error)"=w375) -> ("error out"=w377:errorcluster)  [unwired: 5 in, 1 out]
        n136 = case shown="\"Stopped\"" w378 {
          tunnel: [w385 w388] -> w380
          tunnel: w377 -> [w385 w387]
          tunnel: w374 -> [_ w386]
          frame Default {
          }
          frame "Stopped" {
            n137 = call <vilib>:"Destroy.vi"("error in (no error)"=w387, "SMO"=w386) -> ("error out"=w388:errorcluster)  [unwired: 9 in]
          }
        }
        n138 = call <vilib>:"Add State(s) to Queue__jki_lib_state_machine.vi"("State(s) in (\"\")"=w384) -> ("States Out"=w383:string)  [unwired: 14 in]
      }
      frame "SMO: Hide Instrument UI" {
        # "Do not put any code in this frame.\n(It is a separator no-op. You can make a copy of this frame to create a new Macro frame)"
        n139 = Unbundle By Name(w396) -> ("Instrument UI.lvclass"=w394:refnum<class "Instrument UI.lvclass">)
        n140 = call <vilib>:"GetState.vi"("error in (no error)"=w392, "SMO"=w394) -> ("error out"=w390:errorcluster, "SMO State"=w389:T1, "SMO out"=w393:refnum<class "Instrument UI.lvclass">)  [unwired: 7 in]
        n141 = call <vilib>:"Clear Errors.vi"("error in (no error)"=w390) -> ("error out"=w391:errorcluster)  [unwired: 5 in, 1 out]
        n142 = case shown="Default" w389 {
          tunnel: [w400 w403] -> w395
          tunnel: w393 -> [_ w402]
          tunnel: w391 -> [w400 w401]
          frame Default {
          }
          frame "Started" {
            n143 = call <vilib>:"Hide.vi"("error in (no error)"=w401, "SMO.UI"=w402) -> ("error out"=w403:errorcluster)  [unwired: 8 in, 1 out]
          }
        }
        n144 = call <vilib>:"Add State(s) to Queue__jki_lib_state_machine.vi"("State(s) in (\"\")"=w399) -> ("States Out"=w398:string)  [unwired: 14 in]
      }
      frame "SMO: Stop Instrument UI" {
        # "Do not put any code in this frame.\n(It is a separator no-op. You can make a copy of this frame to create a new Macro frame)"
        n145 = Unbundle By Name(w410) -> ("Instrument UI.lvclass"=w405:refnum<class "Instrument UI.lvclass">)
        n146 = call <vilib>:"GetState.vi"("error in (no error)"=w409, "SMO"=w405) -> ("error out"=w408:errorcluster, "SMO State"=w406:T1, "SMO out"=w404:refnum<class "Instrument UI.lvclass">)  [unwired: 7 in]
        n147 = call <vilib>:"Clear Errors.vi"("error in (no error)"=w408) -> ("error out"=w407:errorcluster)  [unwired: 5 in, 1 out]
        n148 = case shown="\"Created\", \"Started\"" w406 {
          tunnel: [w415 w418] -> w411
          tunnel: w404 -> [_ w417]
          tunnel: w407 -> [w415 w416]
          frame Default {
          }
          frame "Created", "Started" {
            n149 = call <vilib>:"Stop.vi"("error in (no error)"=w416, "SMO"=w417) -> ("error out"=w418:errorcluster)  [unwired: 8 in, 1 out]
          }
        }
        n150 = call <vilib>:"Add State(s) to Queue__jki_lib_state_machine.vi"("State(s) in (\"\")"=w414) -> ("States Out"=w413:string)  [unwired: 14 in]
      }
      frame "SMO: Stop Instrument" {
        # "Do not put any code in this frame.\n(It is a separator no-op. You can make a copy of this frame to create a new Macro frame)"
        n151 = Unbundle By Name(w425) -> ("Instrument.lvclass"=w420:refnum<class "Instrument.lvclass">)
        n152 = call <vilib>:"GetState.vi"("error in (no error)"=w424, "SMO"=w420) -> ("error out"=w423:errorcluster, "SMO State"=w421:T1, "SMO out"=w419:refnum<class "Instrument.lvclass">)  [unwired: 7 in]
        n153 = call <vilib>:"Clear Errors.vi"("error in (no error)"=w423) -> ("error out"=w422:errorcluster)  [unwired: 5 in, 1 out]
        n154 = case shown="\"Created\", \"Started\"" w421 {
          tunnel: [w430 w433] -> w426
          tunnel: w419 -> [_ w432]
          tunnel: w422 -> [w430 w431]
          frame Default {
          }
          frame "Created", "Started" {
            n155 = call <vilib>:"Stop.vi"("error in (no error)"=w431, "SMO"=w432) -> ("error out"=w433:errorcluster)  [unwired: 8 in, 1 out]
          }
        }
        n156 = call <vilib>:"Add State(s) to Queue__jki_lib_state_machine.vi"("State(s) in (\"\")"=w429) -> ("States Out"=w428:string)  [unwired: 14 in]
      }
      frame "SMO: Destroy Instrument UI" {
        # "Do not put any code in this frame.\n(It is a separator no-op. You can make a copy of this frame to create a new Macro frame)"
        n157 = Unbundle By Name(w440) -> ("Instrument UI.lvclass"=w439:refnum<class "Instrument UI.lvclass">)
        n158 = call <vilib>:"GetState.vi"("error in (no error)"=w437, "SMO"=w439) -> ("error out"=w436:errorcluster, "SMO State"=w434:T1, "SMO out"=w438:refnum<class "Instrument UI.lvclass">)  [unwired: 7 in]
        n159 = call <vilib>:"Clear Errors.vi"("error in (no error)"=w436) -> ("error out"=w435:errorcluster)  [unwired: 5 in, 1 out]
        n160 = case shown="Default" w434 {
          tunnel: w435 -> [w445 w448]
          tunnel: [w445 w447] -> w441
          tunnel: w438 -> [_ w446]
          frame Default {
          }
          frame "Stopped" {
            n161 = call <vilib>:"Destroy.vi"("error in (no error)"=w448, "SMO"=w446) -> ("error out"=w447:errorcluster)  [unwired: 9 in]
          }
        }
        n162 = call <vilib>:"Add State(s) to Queue__jki_lib_state_machine.vi"("State(s) in (\"\")"=w444) -> ("States Out"=w443:string)  [unwired: 14 in]
      }
      frame "---------- Splash ----------" {
        # "Template Separator\n(You can make a copy of, or modify, this frame)"
        n163 = call <vilib>:"Add State(s) to Queue__jki_lib_state_machine.vi"("State(s) in (\"\")"=w453) -> ("States Out"=w452:string)  [unwired: 14 in]
      }
      frame "Splash: Set Status" {
        # "Your code here.\n(You can make a copy of, or modify, this frame)"
        n164 = property on="Splash Status" class="Str"(error in=w456, "Value"=w457) -> (error out=w455:errorcluster)  [unwired: 1 in, 1 out]
        n165 = call <vilib>:"Add State(s) to Queue__jki_lib_state_machine.vi"("State(s) in (\"\")"=w460) -> ("States Out"=w459:string)  [unwired: 14 in]
      }
      frame "Splash: 2" {
        # "Your code here.\n(You can make a copy of, or modify, this frame)"
        n166 = call <vilib>:"Add State(s) to Queue__jki_lib_state_machine.vi"("State(s) in (\"\")"=w465) -> ("States Out"=w464:string)  [unwired: 14 in]
      }
    }
  }
  "error out" <- w2
